vi "Host Main.vi"   [LabVIEW 2018]
doc: "This VI is the launcher for the application. It performs and actions required to run before the modules are launched and closes these actions out at application close. All modules are run in parallel and communicate to each other using a communications queue"
uses:
  User Event/User Event Stop FGV Action.ctl
  Modules/Controller (Host)/Controller (Host).lvlib
  Modules/Error Handler/Error Handler.lvlib
  Modules/File IO/File IO.lvlib
  Modules/Testing UI 1/Testing UI 1.lvlib
  Modules/Testing UI 2/Testing UI 2.lvlib
  Modules/Testing UI 3/Testing UI 3.lvlib
  Modules/UDP Writer/PC UDP Writer.lvlib
  Modules/UDP Reader/PC UDP Reader.lvlib
  Modules/Fuel Farm/Fuel Farm.lvlib
panel:
  # "HOST MAIN"
  # "This VI is the launcher for the application. It performs and actions required to run before the modules are launched and closes these actions out at application close. All modules are run in parallel and communicate to each other using a communications queue"
types:
  T1 = typedef "User Event Stop FGV Action.ctl" = enum16{"Get", "Create", "Destroy"}
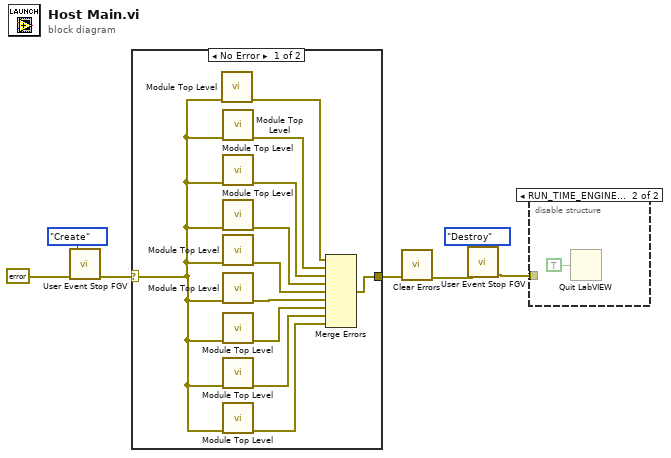
[diagram p0: block diagram]
diagram:
  n1 = call "User Event Stop FGV.vi"("error in (no error)"=errorcluster {"status"=FALSE, "code"=0, "source"=""} ("error in"), "Action (Get)"=User_Event_Stop_FGV_Action."Create") -> ("error out"=w1:errorcluster)  [unwired: 8 in, 1 out]
  n2 = case shown="No Error" w1 {
    selector: w1 -> [w9 w19]
    tunnel: [w18 w19] -> w5
    frame No Error {
      n3 = call "Module Top Level.vi"("error in"=w9) -> ("error out"=w8:errorcluster)  [unwired: 10 in]
      n4 = call "Module Top Level.vi"("error in (no error)"=w9) -> ("error out"=w16:errorcluster)  [unwired: 10 in]
      n5 = call "Module Top Level.vi"("error in (no error)"=w9) -> ("error out"=w17:errorcluster)  [unwired: 10 in]
      n6 = call "Module Top Level.vi"("error in (no error)"=w9) -> ("error out"=w15:errorcluster)  [unwired: 10 in]
      n7 = call "Module Top Level.vi"("error in"=w9) -> ("error out"=w11:errorcluster)  [unwired: 10 in]
      n8 = call "Module Top Level.vi"("error in"=w9) -> ("error out"=w10:errorcluster)  [unwired: 10 in]
      n9 = call "Module Top Level.vi"("error in"=w9) -> ("error out"=w14:errorcluster)  [unwired: 10 in]
      n10 = call "Module Top Level.vi"("error in"=w9) -> ("error out"=w13:errorcluster)  [unwired: 10 in]
      n11 = call "Module Top Level.vi"("error in"=w9) -> ("error out"=w12:errorcluster)  [unwired: 10 in]
      n12 = Merge Errors(w8, w16, w17, w15, w11, w10, w14, w13, w12) -> (w18:errorcluster)
    }
    frame Error {
    }
  }
  n13 = call <vilib>:"Clear Errors.vi"("error in (no error)"=w5) -> ("error out"=w4:errorcluster)  [unwired: 5 in, 1 out]
  n14 = call "User Event Stop FGV.vi"("error in (no error)"=w4, "Action (Get)"=User_Event_Stop_FGV_Action."Destroy") -> ("error out"=w2:errorcluster)  [unwired: 8 in, 1 out]
  n15 = disable-structure shown="RUN_TIME_ENGINE==True" {
    disable-tunnel: w2 -> [_ _]
    frame condition #0 (active) {
    }
    frame condition #1 {
      n16 = Quit LabVIEW(quit? (T)=TRUE) -> ()
    }
  }
